vi "ReadIniFile.vi"(0 "key":string="FrontPanelPosition") -> (1 "value":string, 2 "found?":bool)   [LabVIEW 2014]
uses:
  <vilib>/Utility/config.llb/Read Key (String).vi
  <vilib>/Utility/config.llb/NI_LVConfig.lvlib
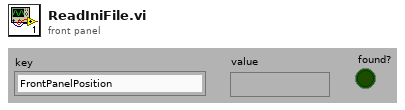
[diagram p1: front panel]
types:
  T1 = typedef "NI_LVConfig.lvlib/Config Data RefNum.ctl" = refnum<k1>
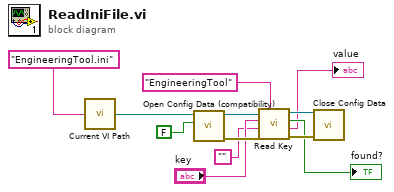
[diagram p0: block diagram]
diagram:
  n1 = call "Current VI Path.vi"("file name"="EngineeringTool.ini" ("name or relative path")) -> ("Path for file"=w1:path)
  n2 = call <vilib>:"Open Config Data (compatibility).vi"("create file if necessary (T)"=FALSE ("create file if necessary? (T)"), "configuration file path"=w1) -> ("error out"=w9:errorcluster, "refnum"=w12:T1)  [unwired: 7 in, 1 out]
  n3 = call-poly <vilib>:"Read Key.vi"("section"="EngineeringTool", "error in (no error)"=w9, "default value"="", "key"="key", "refnum"=w12) -> ("error out"=w7:errorcluster, "value"=→"value":string, "found?"=→"found?":bool, "refnum out"=w8:T1)  [unwired: 3 in]
  n4 = call <vilib>:"Close Config Data.vi"("error in (no error)"=w7, "refnum"=w8) -> ()  [unwired: 8 in, 2 out]
